vi "host.vi"() -> ()   [LabVIEW 2020]
uses:
  b4957acc-33c7-4f51-b6c8-be02e890b770.vi
  <vilib>/Array/Sort 2D Array - Pop Stack.vi
  <vilib>/Array/Sort 2D Array - Push Stack.vi
  b4957acc-33c7-4f51-b6c8-be02e890b770.vi/269d4b3b-47f5-49e3-8884-44851e4dd9d5.vi
  b4957acc-33c7-4f51-b6c8-be02e890b770.vi/6d99389c-673d-4efb-bf33-19b32bcf4cf8.vi
  <vilib>/FPGAPlugInAG/cRIO-9035/niLvFpga_Open_cRIO-9035.vi
  <vilib>/FPGAPlugInAG/cRIO-9035/niLvFpga_Reset_cRIO-9035.vi
  <vilib>/Utility/error.llb/Error Cluster From Error Code.vi
  <vilib>/rvi/errors/niLvFpgaAdjustHostInterfaceError.vi
  <vilib>/FPGAPlugInAG/cRIO-9035/niLvFpga_Run_cRIO-9035.vi
  <vilib>/FPGAPlugInAG/cRIO-9035/niLvFpga_Close_cRIO-9035.vi
  <vilib>/rvi/interface/nirviOpenFPGA/nirviOpenFPGA.xnode
  FPGA Bitfiles/project_FPGATarget_target_eh4G3bHM0Kw.lvbitx
  target.vi
  <vilib>/rvi/interface/nirviMethod/nirviMethod.xnode
  <vilib>/rvi/interface/nirviReadWriteControl/nirviReadWriteControl.xnode
  <vilib>/rvi/interface/nirviCloseFPGA/nirviCloseFPGA.xnode
  <vilib>/Analysis/NI_AALBase.lvlib
  <vilib>/FPGAPlugInAG/cRIO-9035/niLvFpga_StartFifo_cRIO-9035.vi
  <vilib>/rvi/errors/niLvFpgaMergeErrorWithErrorCode.vi
  <vilib>/FPGAPlugInAG/cRIO-9035/niLvFpga_WriteFifo_cRIO-9035.vi
  <vilib>/FPGAPlugInAG/cRIO-9035/niLvFpga_ReadFifo_cRIO-9035.vi
  NiFpgaLv.dll
panel:
  out "Data":sgl[](array[numeric])
  out "error out":errorcluster
  out "Timed Out? FIFO out index":bool
  out "Timed Out? FIFO out IMG":bool
  out "Timed Out? FIFO out REAL":bool
  out "Timed Out? FIFO in REAL":bool
  out "Timed Out? FIFO in IMG":bool
  out "IMG sorted signal":sgl[](graph)
  out "index values":i32[](array[numeric])
  out "sorted 2D array":sgl[][](array[numeric])
  out "input data":sgl[](graph)
  out "sort time (ms)":dbl
  out "Elements Remaining":u32
  out "Real sorted signal":sgl[](graph)
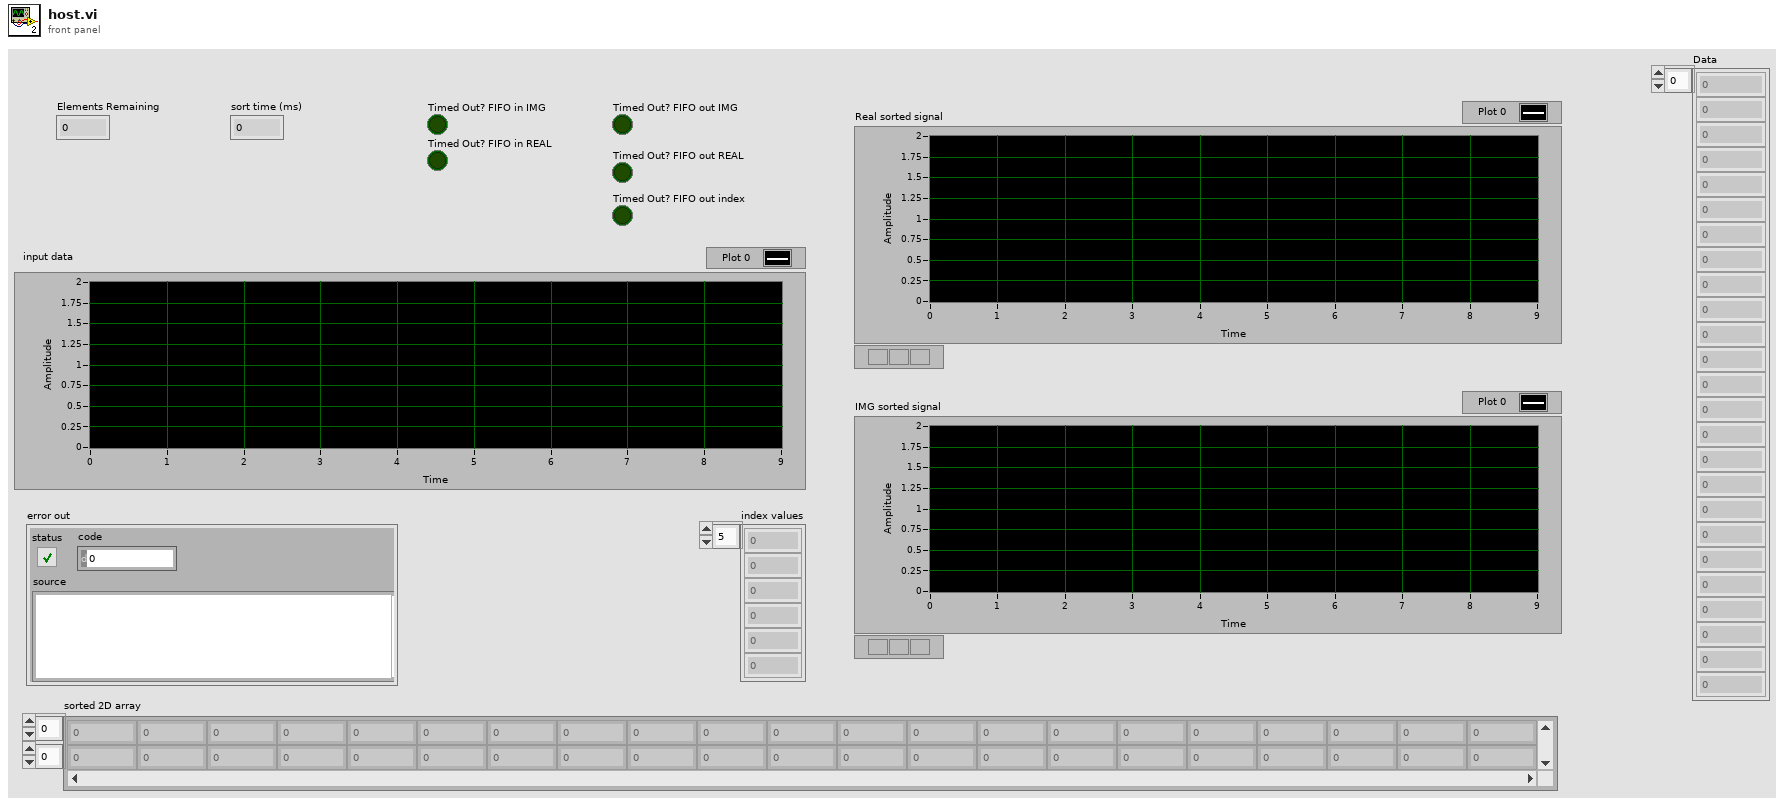
[diagram p1: front panel]
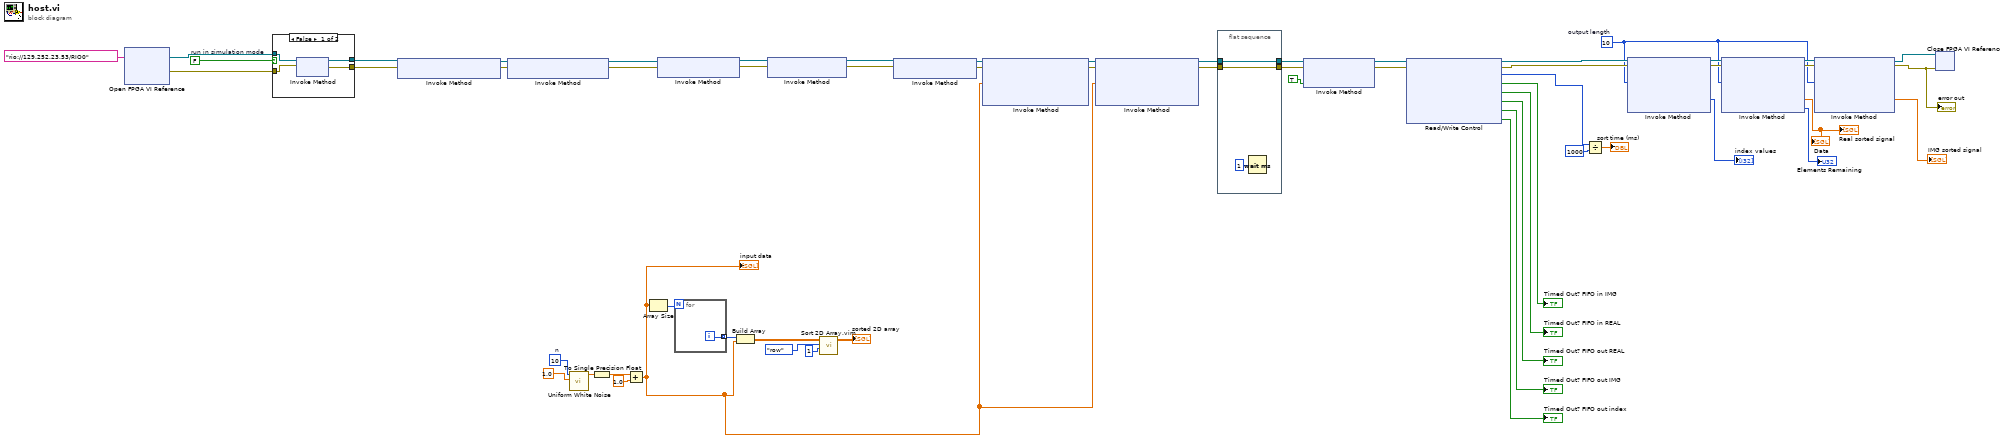
[diagram p0: block diagram]
diagram:
  w7 = FALSE  # run in simulation mode
  w37 = 10  # n
  w24 = u32 10  # output length
  n1 = xnode "Open FPGA VI Reference"("resource name"=tag "rio://129.252.23.53/RIO0") -> ("FPGA VI Reference Out"=w6:refnum<k20>, "error out"=w5:errorcluster)  [unwired: 1 in]
  n2 = case shown="False" w7 {
    tunnel: w6 -> [w62 w63]
    tunnel: w5 -> [w61 w64]
    tunnel: [w60 w63] -> w4
    tunnel: [w59 w64] -> w3
    frame False {
      n3 = xnode "Invoke Method"("FPGA VI Reference In"=w62, "error in"=w61) -> ("FPGA VI Reference Out"=w60:refnum<k20>, "error out"=w59:errorcluster)
    }
    frame True {
    }
  }
  n4 = xnode "Invoke Method"("FPGA VI Reference In"=w4, "error in"=w3) -> ("FPGA VI Reference Out"=w34:refnum<k20>, "error out"=w33:errorcluster)
  n5 = xnode "Invoke Method"("FPGA VI Reference In"=w34, "error in"=w33) -> ("FPGA VI Reference Out"=w19:refnum<k20>, "error out"=w18:errorcluster)
  n6 = call <vilib>:"Uniform White Noise.vi"("amplitude"=1.0, "samples"=w37) -> ("uniform white noise"=w36:dbl[])  [unwired: 8 in, 1 out]
  n7 = To Single Precision Float(number=w36) -> (single precision float=w35:sgl[])
  n8 = Add(x=w35, y=sgl 1.0 ("amplitude")) -> (x+y=w2:sgl[])
  "input data" <- w2
  n9 = Array Size(array=w2) -> (size(s)=w42:i32)
  n10 = xnode "Invoke Method"("FPGA VI Reference In"=w19, "error in"=w18) -> ("FPGA VI Reference Out"=w17:refnum<k20>, "error out"=w22:errorcluster)
  n11 = for {
    N: w42 -> [_]
    tunnel: [w65] -> w41 mode=indexing
    i -> [w65]
  }
  n12 = Build Array(w41, w2) -> (w40:sgl[][])
  n13 = xnode "Invoke Method"("FPGA VI Reference In"=w17, "error in"=w22) -> ("FPGA VI Reference Out"=w21:refnum<k20>, "error out"=w20:errorcluster)
  n14 = call "Sort 2D Array.vim"("index"=1, "dimension to index (column)"=enum16{"column", "row"}."row", "2D array"=w40) -> ("sorted 2D array"=→"sorted 2D array":sgl[][])  [unwired: 7 in, 1 out]
  n15 = xnode "Invoke Method"("FPGA VI Reference In"=w21, "error in"=w20) -> ("FPGA VI Reference Out"=w32:refnum<k20>, "error out"=w31:errorcluster)
  n16 = xnode "Invoke Method"("FPGA VI Reference In"=w32, "error in"=w31, "Data"=w2) -> ("FPGA VI Reference Out"=w30:refnum<k20>, "error out"=w29:errorcluster)  [unwired: 1 in, 1 out]
  n17 = xnode "Invoke Method"("FPGA VI Reference In"=w30, "error in"=w29, "Data"=w2) -> ("FPGA VI Reference Out"=w10:refnum<k20>, "error out"=w8:errorcluster)  [unwired: 1 in, 1 out]
  n18 = flat-sequence {
    tunnel: [w67] -> w11
    tunnel: w10 -> [w67]
    tunnel: [w66] -> w9
    tunnel: w8 -> [w66]
    frame #0 {
      n19 = Wait (ms)(milliseconds to wait=u32 1) -> ()  [unwired: 1 out]
    }
  }
  n20 = xnode "Invoke Method"("FPGA VI Reference In"=w11, "error in"=w9, "Wait Until Done (F)"=TRUE) -> ("FPGA VI Reference Out"=w55:refnum<k20>, "error out"=w54:errorcluster)
  n21 = xnode "Read/Write Control"("FPGA VI Reference In"=w55, "error in"=w54) -> ("FPGA VI Reference Out"=w49:refnum<k20>, "error out"=w47:errorcluster, "sort time (us)"=w53:u32, "Timed Out? FIFO in IMG"=→"Timed Out? FIFO in IMG":bool, "Timed Out? FIFO in REAL"=→"Timed Out? FIFO in REAL":bool, "Timed Out? FIFO out REAL"=→"Timed Out? FIFO out REAL":bool, "Timed Out? FIFO out IMG"=→"Timed Out? FIFO out IMG":bool, "Timed Out? FIFO out index"=→"Timed Out? FIFO out index":bool)
  n22 = Divide(x=w53, y=u32 1000) -> (x/y=→"sort time (ms)":dbl)
  n23 = xnode "Invoke Method"("FPGA VI Reference In"=w49, "error in"=w47, "Number of Elements"=w24) -> ("FPGA VI Reference Out"=w48:refnum<k20>, "error out"=w46:errorcluster, "Data"=→"index values":i32[])  [unwired: 1 in, 1 out]
  n24 = xnode "Invoke Method"("FPGA VI Reference In"=w48, "error in"=w46, "Number of Elements"=w24) -> ("FPGA VI Reference Out"=w28:refnum<k20>, "error out"=w27:errorcluster, "Data"=→"Real sorted signal" →"Data":sgl[], "Elements Remaining"=→"Elements Remaining":u32)  [unwired: 1 in]
  n25 = xnode "Invoke Method"("FPGA VI Reference In"=w28, "error in"=w27, "Number of Elements"=w24) -> ("FPGA VI Reference Out"=w26:refnum<k20>, "error out"=w25:errorcluster, "Data"=→"IMG sorted signal":sgl[])  [unwired: 1 in, 1 out]
  "error out" <- w25
  n26 = xnode "Close FPGA VI Reference"("FPGA VI Reference In"=w26, "error in"=w25) -> ()  [unwired: 1 out]
